vi "Read Configuration Data.vi"(8 "error in (no error)":errorcluster) -> (0 "error out":errorcluster, 3 "MHL Configuration":T1)   [LabVIEW 2015]
uses:
  controls/MHL Configuration.ctl
  Boiler System Globals.vi
  <vilib>/Utility/config.llb/NI_LVConfig.lvlib
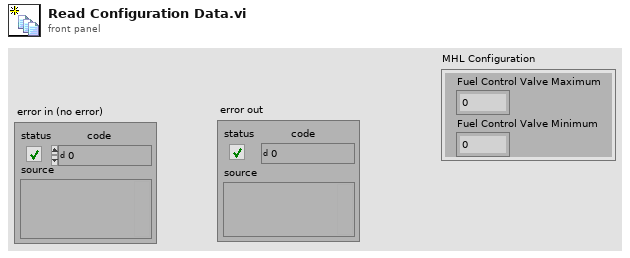
[diagram p1: front panel]
types:
  T1 = typedef "MHL Configuration.ctl" = cluster{"Fuel Control Valve Maximum":dbl, "Fuel Control Valve Minimum":dbl}
  T2 = typedef "NI_LVConfig.lvlib/Config Data RefNum.ctl" = refnum<k1>
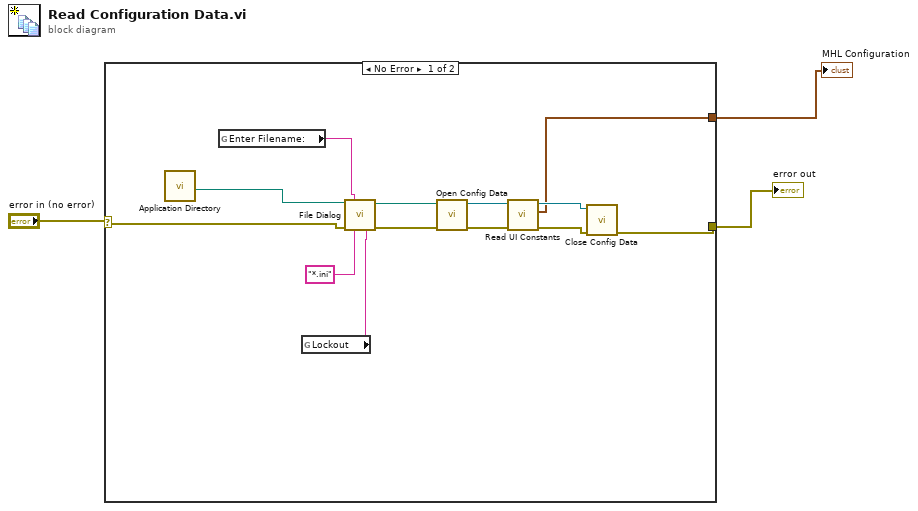
[diagram p0: block diagram]
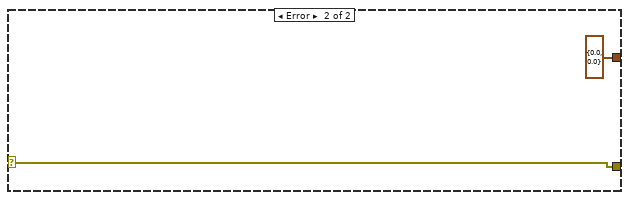
[diagram p2: hidden frame]
diagram:
  n1 = case shown="No Error" "error in (no error)" {
    selector: "error in (no error)" -> [w5 w18]
    tunnel: [w7 w18] -> w2
    tunnel: [w6 T1 {"Fuel Control Valve Maximum"=0.0, "Fuel Control Valve Minimum"=0.0} ("MHL Configuration")] -> w1
    frame No Error {
      n2 = call <vilib>:"Application Directory.vi"() -> ("Application Directory"=w4:path)
      n3 = global read "Boiler System Globals.vi" "Enter Filename:"() -> (w14:string)
      n4 = global read "Boiler System Globals.vi" "Lockout"() -> (w15:string)
      n5 = call "File Dialog"("start path"=w4, "prompt"=w14, "error in"=w5, "pattern (all files)"="*.ini", "pattern label"=w15) -> ("selected path"=w13:path, "error out"=w12:errorcluster)  [unwired: 7 in, 2 out]
      n6 = call <vilib>:"Open Config Data.vi"("error in (no error)"=w12, "configuration file path"=w13) -> ("error out"=w11:errorcluster, "refnum"=w10:T2)  [unwired: 7 in, 1 out]
      n7 = call "Read UI Constants.vi"("error in (no error)"=w11, "CFG File Refnum"=w10) -> ("error out"=w8:errorcluster, "MHL Configuration"=w6:T1, "CFG File Refnum out"=w9:T2)  [unwired: 7 in]
      n8 = call <vilib>:"Close Config Data.vi"("error in (no error)"=w8, "refnum"=w9) -> ("error out"=w7:errorcluster)  [unwired: 8 in, 1 out]
    }
    frame Error {
    }
  }
  "error out" <- w2
  "MHL Configuration" <- w1
